vi "Load Section - Paths.vi"(8 "error in (no error)":errorcluster, 11 "JSON string":string) -> (0 "error out":errorcluster, 3 "Class data":refnum<class "Settings Service.lvclass">)   [LabVIEW 2026, in "Settings Service.lvclass"]
uses:
  Settings Service.lvclass
  Settings Service.lvclass/Settings Service.ctl
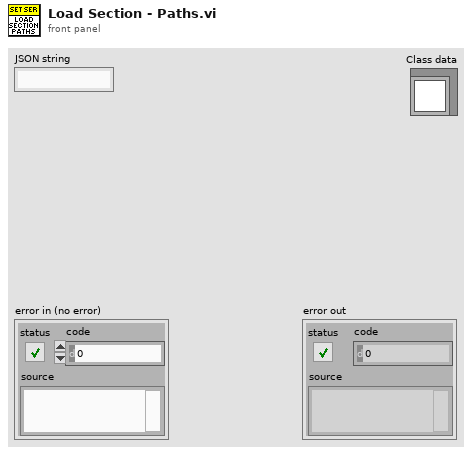
[diagram p1: front panel]
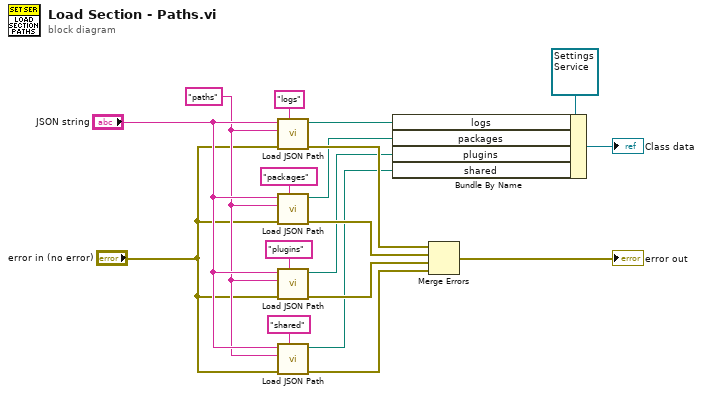
[diagram p0: block diagram]
diagram:
  w4 = "paths" ("Section")
  n1 = call "Load JSON Path.vi"("Element"="logs", "error in (no error)"="error in (no error)", "Section"=w4, "JSON string"="JSON string") -> ("error out"=w16:errorcluster, "value"=w12:path)  [unwired: 6 in]
  n2 = call "Load JSON Path.vi"("Element"="packages", "error in (no error)"="error in (no error)", "Section"=w4, "JSON string"="JSON string") -> ("error out"=w15:errorcluster, "value"=w11:path)  [unwired: 6 in]
  n3 = call "Load JSON Path.vi"("Element"="plugins", "error in (no error)"="error in (no error)", "Section"=w4, "JSON string"="JSON string") -> ("error out"=w8:errorcluster, "value"=w7:path)  [unwired: 6 in]
  n4 = call "Load JSON Path.vi"("Element"="shared", "error in (no error)"="error in (no error)", "Section"=w4, "JSON string"="JSON string") -> ("error out"=w2:errorcluster, "value"=w1:path)  [unwired: 6 in]
  n5 = Bundle By Name(cluster=refnum<class "Settings Service.lvclass"> refnum ("Settings Service.lvclass"), "logs"=w12, "packages"=w11, "plugins"=w7, "shared"=w1) -> (→"Class data":refnum<class "Settings Service.lvclass">)
  n6 = Merge Errors(w16, w15, w8, w2) -> (→"error out":errorcluster)
